vi "Chapter-Two.vi"() -> ()   [LabVIEW 2023]
uses:
  <vilib>/ActorFramework/Message Enqueuer/Message Enqueuer.lvclass
  MQTT-Server/MQTT-Server/MQTT-Server.lvclass
  C:/Program Files/National Instruments/LabVIEW 2023/vi.lib/ActorFramework/Actor/Actor.lvclass
  MQTT-Client/MQTT-Client/MQTT-Client.lvclass
  MQTT-Client/MQTT-Client/MQTT-Client.lvclass/MQTT-Client.ctl
  <vilib>/ActorFramework/Message Enqueuer/Message Enqueuer.lvclass/Message Enqueuer.ctl
  MQTT-Client/MQTT-Client Messages/Schedule Msg/Schedule Msg.lvclass/Schedule Msg.ctl
  MQTT-Client/MQTT-Client Messages/Payload Msg/Payload Msg.lvclass/Payload Msg.ctl
  <vilib>/ActorFramework/Message Enqueuer/Enqueue.vi
  <vilib>/ActorFramework/Stop Msg/Stop Msg.lvclass
  C:/Program Files/National Instruments/LabVIEW 2023/vi.lib/ActorFramework/Message/Message.lvclass
  MQTT-Client/MQTT-Client Messages/Schedule Msg/Schedule Msg.lvclass
  MQTT-Client/MQTT-Client Messages/Payload Msg/Payload Msg.lvclass
  <vilib>/ActorFramework/Message Priority Queue/Priority Enqueue.vi
  <vilib>/ActorFramework/Actor/Actor.lvclass
panel:
  out "Actor's Enqueuer":refnum<class "Message Enqueuer.lvclass">
  out "PayLoadSize":i32 min=0 step=1 format="%.0pbytes"
  in  "Payload":string
  in  "Schedule":i32=100 min=0 step=1 format="%.0p ms"
  in  "Client No.":i32 min=0 step=1
  in  "Server":bool
  in  "Stop":bool
  # "Client"
  # "Server"
  # "Demo"
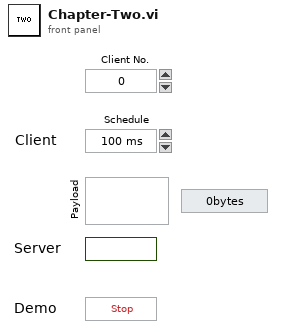
[diagram p1: front panel]
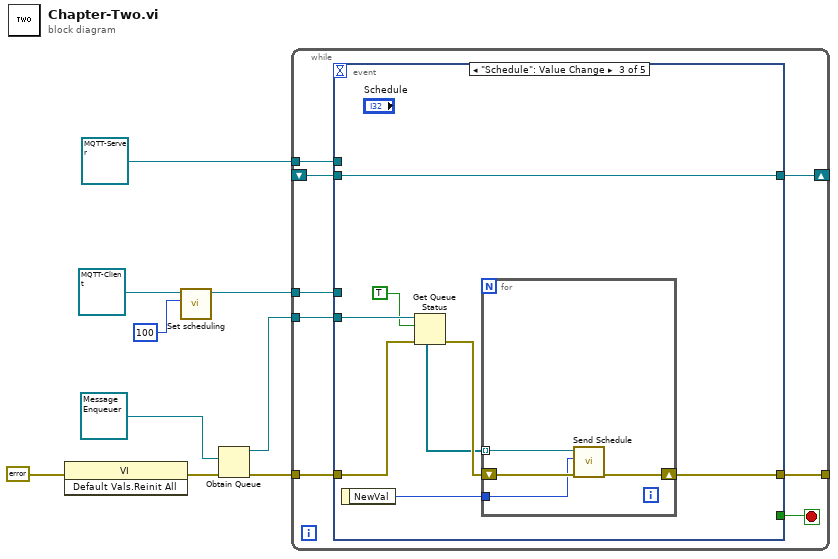
[diagram p0: block diagram]
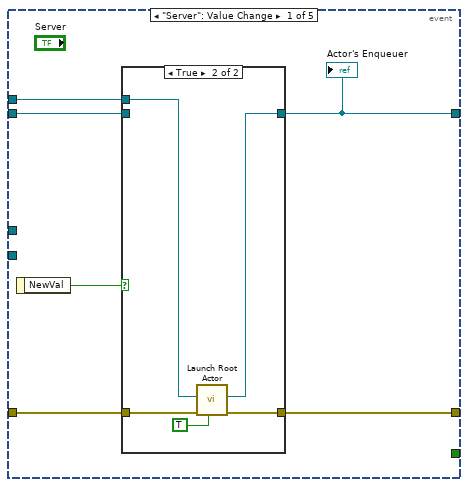
[diagram p2: hidden frame]
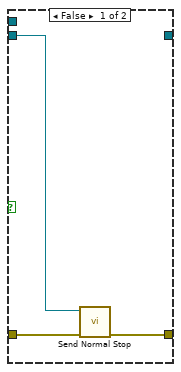
[diagram p3: hidden frame]
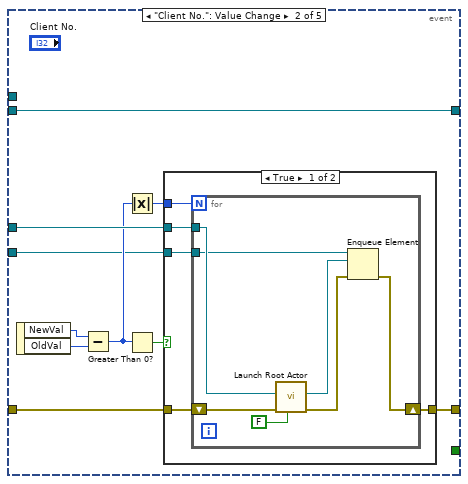
[diagram p4: hidden frame]
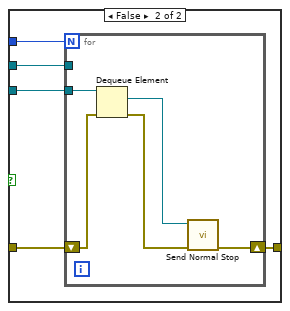
[diagram p5: hidden frame]
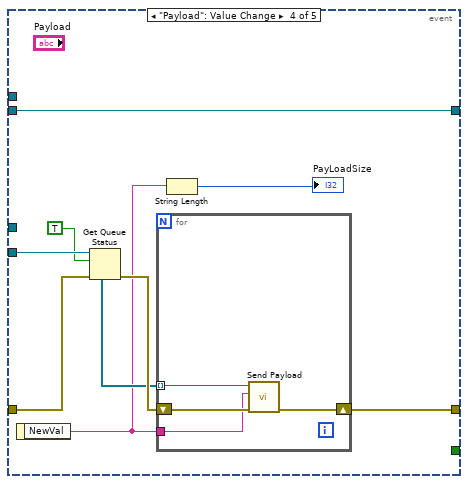
[diagram p6: hidden frame]
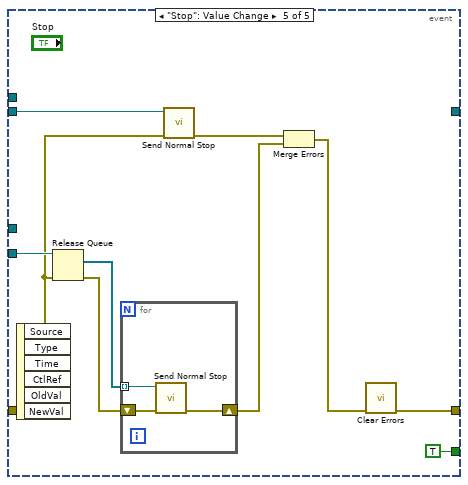
[diagram p7: hidden frame]
diagram:
  n1 = invoke class="VI" method="Default Vals.Reinit All"(error in=errorcluster {"status"=FALSE, "code"=0, "source"=""} ("error in (no error)")) -> (error out=w2:errorcluster)  [unwired: 2 in, 2 out]
  n2 = call "Set scheduling.vi"("scheduling"=100, "MQTT-Client in"=refnum<class "MQTT-Client.lvclass"> refnum ("MQTT-Client.lvlib:MQTT-Client.lvclass")) -> ("MQTT-Client out"=w5:refnum<class "MQTT-Client.lvclass">)  [unwired: 8 in, 1 out]
  n3 = Obtain Queue(element data type=refnum<class "Message Enqueuer.lvclass"> refnum ("Actor's Enqueuer"), error in (no error)=w2) -> (queue out=w1:refnum<queue>, error out=w8:errorcluster)  [unwired: 3 in, 1 out]
  n4 = while {
    tunnel: refnum<class "MQTT-Server.lvclass"> refnum ("MQTT-Server.lvlib:MQTT-Server.lvclass") -> [w17]
    tunnel: w5 -> [w16]
    tunnel: w8 -> [w15]
    tunnel: [w14] -> _
    shift-right: [w13] -> _
    shift-left: _ -> [w12]
    tunnel: w1 -> [w11]
    stop <- w10 stop-if-true
    n5 = event shown="[2] \"Schedule\": Value Change" {
      selector: _ -> [_ _ _ _ _]
      dyn-events: _ -> [_ _ _ _ _]
      timeout: _ -> [_ _ _ _ _]
      tunnel: w17 -> [w23 _ _ _ _]
      tunnel: w16 -> [_ w38 _ _ _]
      tunnel: w15 -> [w22 w37 w70 w83 w95]
      tunnel: [w21 w33 w66 w79 w90] -> w14
      tunnel: [w20 w41 w71 w84 _] -> w13
      tunnel: w12 -> [w19 w41 w71 w84 w94]
      tunnel: w11 -> [_ w34 w69 w82 w98]
      tunnel: [_ _ _ _ TRUE] -> w10
      event "Server": Value Change {
        n6 = event-data() -> ("NewVal"=w18:bool)  [unwired: 1 in]
        n7 = case shown="True" w18 {
          tunnel: w23 -> [_ w31]
          tunnel: w22 -> [w25 w30]
          tunnel: [w24 w28] -> w21
          tunnel: [_ w27] -> w20
          tunnel: w19 -> [w26 _]
          frame False {
            n8 = call <vilib>:"Send Normal Stop.vi"("error in (no error)"=w25, "Message Enqueuer"=w26) -> ("error out"=w24:errorcluster)  [unwired: 9 in]
          }
          frame True {
            n9 = call <vilib>:"Launch Root Actor.vi"("Open Actor Core front panel? (F)"=TRUE, "error in (no error)"=w30, "Actor"=w31) -> ("error out"=w28:errorcluster, "Actor's Enqueuer"=w27:refnum<class "Message Enqueuer.lvclass">)  [unwired: 7 in]
          }
        }
        "Actor's Enqueuer" <- w20
      }
      event "Client No.": Value Change {
        n10 = event-data() -> ("NewVal"=w40:i32, "OldVal"=w39:i32)  [unwired: 1 in]
        n11 = Subtract(x=w40, y=w39) -> (x-y=w36:i32)
        n12 = Absolute Value(x=w36) -> (abs(x)=w35:i32)
        n13 = Greater Than 0?(x=w36) -> (x > 0?=w32:bool)
        n14 = case shown="True" w32 {
          tunnel: w38 -> [w46 w58]
          tunnel: w37 -> [w45 w57]
          tunnel: w35 -> [w44 w56]
          tunnel: w34 -> [w43 w55]
          tunnel: [w42 w54] -> w33
          frame True {
            n15 = for {
              N: w44 -> [_]
              tunnel: w46 -> [w52]
              shift-right: [w47] -> w42
              shift-left: w45 -> [w53]
              tunnel: w43 -> [w50]
              n16 = call <vilib>:"Launch Root Actor.vi"("Open Actor Core front panel? (F)"=FALSE, "error in (no error)"=w53, "Actor"=w52) -> ("error out"=w49:errorcluster, "Actor's Enqueuer"=w48:refnum<class "Message Enqueuer.lvclass">)  [unwired: 7 in]
              n17 = Enqueue Element(queue=w50, element=w48, error in (no error)=w49) -> (error out=w47:errorcluster)  [unwired: 1 in, 2 out]
            }
          }
          frame False {
            n18 = for {
              N: w56 -> [_]
              tunnel: w58 -> [_]
              shift-right: [w59] -> w54
              shift-left: w57 -> [w62]
              tunnel: w55 -> [w63]
              n19 = Dequeue Element(queue=w63, error in (no error)=w62) -> (element=w61:refnum<class "Message Enqueuer.lvclass">, error out=w60:errorcluster)  [unwired: 1 in, 2 out]
              n20 = call <vilib>:"Send Normal Stop.vi"("error in (no error)"=w60, "Message Enqueuer"=w61) -> ("error out"=w59:errorcluster)  [unwired: 9 in]
            }
          }
        }
      }
      event "Schedule": Value Change {
        n21 = event-data() -> ("NewVal"=w64:i32)  [unwired: 1 in]
        n22 = Get Queue Status(queue=w69, return elements? (F)=TRUE, error in (no error)=w70) -> (error out=w67:errorcluster, elements=w65:refnum<class "Message Enqueuer.lvclass">[])  [unwired: 6 out]
        n23 = for {
          shift-right: [w74] -> w66
          shift-left: w67 -> [w75]
          tunnel: w65 -> [w73] mode=indexing
          tunnel: w64 -> [w72]
          n24 = call "Send Schedule.vi"("error in (no error)"=w75, "scheduling"=w72, "Message Enqueuer"=w73) -> ("error out"=w74:errorcluster)  [unwired: 7 in, 1 out]
        }
      }
      event "Payload": Value Change {
        n25 = event-data() -> ("NewVal"=w77:string)  [unwired: 1 in]
        n26 = Get Queue Status(queue=w82, return elements? (F)=TRUE, error in (no error)=w83) -> (error out=w80:errorcluster, elements=w78:refnum<class "Message Enqueuer.lvclass">[])  [unwired: 6 out]
        n27 = for {
          shift-right: [w87] -> w79
          shift-left: w80 -> [w88]
          tunnel: w78 -> [w86] mode=indexing
          tunnel: w77 -> [w85]
          n28 = call "Send Payload.vi"("error in (no error)"=w88, "payload"=w85, "Message Enqueuer"=w86) -> ("error out"=w87:errorcluster)  [unwired: 7 in, 1 out]
        }
        n29 = String Length(string=w77) -> (length=→"PayLoadSize":i32)
      }
      event "Stop": Value Change {
        n30 = event-data() -> ()  [unwired: 1 in, 6 out]
        n31 = Release Queue(queue=w98, error in (no error)=w95) -> (remaining elements=w96:refnum<class "Message Enqueuer.lvclass">[], error out=w97:errorcluster)  [unwired: 1 in, 1 out]
        n32 = for {
          tunnel: w96 -> [w100] mode=indexing
          shift-right: [w99] -> w93
          shift-left: w97 -> [w101]
          n33 = call <vilib>:"Send Normal Stop.vi"("error in (no error)"=w101, "Message Enqueuer"=w100) -> ("error out"=w99:errorcluster)  [unwired: 9 in]
        }
        n34 = call <vilib>:"Send Normal Stop.vi"("error in (no error)"=w95, "Message Enqueuer"=w94) -> ("error out"=w92:errorcluster)  [unwired: 9 in]
        n35 = Merge Errors(w92, w93) -> (w91:errorcluster)
        n36 = call <vilib>:"Clear Errors.vi"("error in (no error)"=w91) -> ("error out"=w90:errorcluster)  [unwired: 5 in, 1 out]
      }
    }
  }
